vi "Get Display.vi"(8 "Error In":errorcluster, 11 "Draw Frame In":refnum<class "Draw Frame.lvclass">) -> (0 "Error Out":errorcluster, 2 "Display":refnum<class "Display.lvclass">, 3 "Draw Frame Out":refnum<class "Draw Frame.lvclass">)   [LabVIEW 2021, in "Draw Frame.lvclass"]
uses:
  Draw Frame.lvclass
  <vilib>/Memosfet/myRIO-Neopixel/RT/Display/Display.lvclass
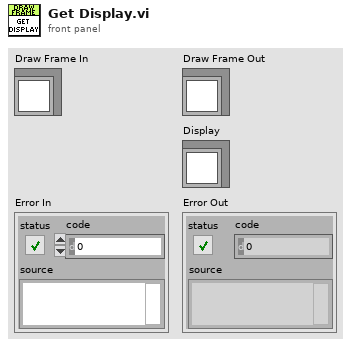
[diagram p1: front panel]
types:
  T1 = typedef "Draw Frame.lvclass/Data.ctl" = cluster{"Display":refnum<class "Display.lvclass">, "FPGA Reference":T2}
  T2 = typedef "Draw Frame.lvclass/FPGA Reference.ctl" = refnum<k20>
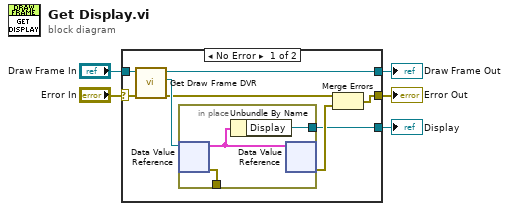
[diagram p0: block diagram]
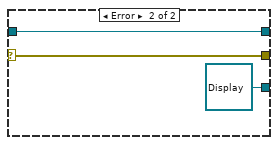
[diagram p2: hidden frame]
diagram:
  n1 = case shown="No Error" "Error In" {
    selector: "Error In" -> [w9 w18]
    tunnel: [w11 w18] -> w2
    tunnel: [w8 w19] -> w4
    tunnel: "Draw Frame In" -> [w10 w19]
    tunnel: [w12 refnum<class "Display.lvclass"> refnum ("Display")] -> w1
    frame No Error {
      n2 = call "Get Draw Frame DVR.vi"("Error In"=w9, "Draw Frame In"=w10) -> ("Error Out"=w6:errorcluster, "DVR"=w7:refnum<data-value>, "Draw Frame Out"=w8:refnum<class "Draw Frame.lvclass">)  [unwired: 7 in]
      n3 = in-place {
        in-place-border: [w14] -> w12
        in-place-border: [w16] -> _
        n4 = in-place-dvr #1(w7) -> (w15:T1, w16:errorcluster)
        n5 = Unbundle By Name(w15) -> ("Display"=w14:refnum<class "Display.lvclass">)
        n6 = in-place-dvr #1(w15) -> (w13:errorcluster)  [unwired: 1 out]
      }
      n7 = Merge Errors(w6, w13) -> (w11:errorcluster)
    }
    frame Error {
    }
  }
  "Draw Frame Out" <- w4
  "Error Out" <- w2
  "Display" <- w1
